vi "Sync Source.vi"() -> ()   [LabVIEW 2011, in "LVH-Toolbox.lvlib" / "LVH-Build-Tools.lvlib"]
doc: "This VI duplicates the install directories folder hierarchy in the source directory and creates hard links in the source directory for each file in the install directory. This VI should be run each time after LabVIEW development, before checking in code."
uses:
  LVH-Build-Tools.lvlib
panel:
  in  "Uninstall and Mass Compile Source?":bool
  out "Deleted Files":path[](array[path])
  out "Added Files":path[](array[path])
  # "Sync Source"
  # "1. Run this VI\n2. When prompted select the config.ini file for the project you are working on.  The config.ini should be in the soure root directory.\n3. This VI will create hard links from for everything in the Install dirctory in the Source Root directory.\n\nNote: Do not open any VI's from the source directory.  All edits should be done in the Install directory to preserve paths."
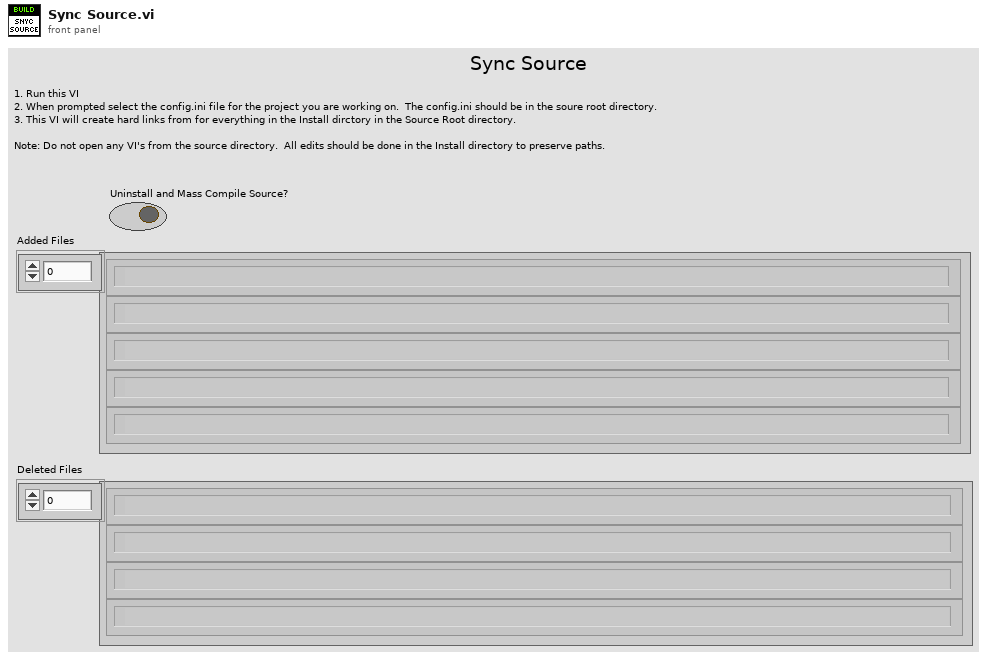
[diagram p1: front panel]
types:
  T1 = typedef "LVH-Toolbox.lvlib/LVH-Build-Tools.lvlib/Configuration.ctl" = cluster{"Source Root":string, "Install Root":string, "Components":string[], "Ignore":string[]}
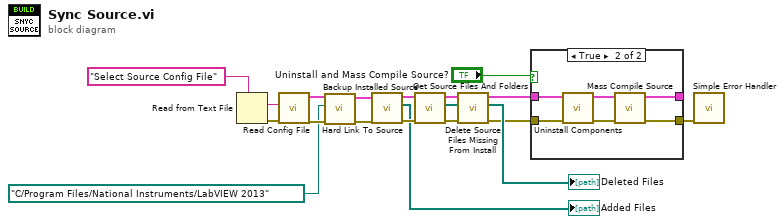
[diagram p0: block diagram]
diagram:
  n1 = Read from Text File(prompt (Open existing file)="Select Source Config File") -> (text=w17:string, error out=w19:errorcluster)  [unwired: 3 in, 2 out]
  n2 = call "Read Config File.vi"("error in (no error)"=w19, "Config File In"=w17) -> ("error out"=w4:errorcluster, "Configuration out"=w5:T1)  [unwired: 8 in]
  n3 = call "Backup Installed Source.vi"("Error In"=w4, "LabVIEW Dir"=path "C:/Program Files/National Instruments/LabVIEW 2013", "Configuration"=w5) -> ("Error Out"=w3:errorcluster, "Configuration"=w2:T1)  [unwired: 7 in]
  n4 = call "Hard Link To Source.vi"("Error In"=w3, "Configuration in"=w2) -> ("Error Out"=w16:errorcluster, "Files Added To Source"=→"Added Files":path[], "Configuration out"=w11:T1)  [unwired: 7 in]
  n5 = call "Get Source Files And Folders.vi"("Error In"=w16, "Configuration"=w11) -> ("Error Out"=w15:errorcluster, "All Source Files"=w13:path[], "Configuration"=w14:T1)  [unwired: 6 in, 1 out]
  n6 = call "Delete Source Files Missing From Install.vi"("Error In"=w15, "Source Files"=w13, "Configuration"=w14) -> ("Error Out"=w9:errorcluster, "Deleted From Souce"=→"Deleted Files":path[], "Configuration"=w7:T1)  [unwired: 6 in]
  n7 = case shown="True" "Uninstall and Mass Compile Source?" {
    tunnel: w9 -> [w20 w22]
    tunnel: [w21 w25] -> _
    tunnel: [w20 w24] -> w8
    tunnel: w7 -> [w21 w23]
    frame False {
    }
    frame True {
      n8 = call "Uninstall Components.vi"("error in (no error)"=w22, "Configuration in"=w23) -> ("error out"=w26:errorcluster, "Configuration out"=w27:T1)  [unwired: 7 in, 1 out]
      n9 = call "Mass Compile Source.vi"("error in (no error)"=w26, "Configuration in"=w27) -> ("error out"=w24:errorcluster, "Configuration out"=w25:T1)  [unwired: 8 in]
    }
  }
  n10 = call <vilib>:"Simple Error Handler.vi"("error in (no error)"=w8) -> ()  [unwired: 4 in, 5 out]
